vi "Min position limit.vi"(8 "error in (no error)":errorcluster, 9 "W/R":enum16{"Write", "Read"}(ring), 10 "Data":i32, 11 "Motor Base in":refnum<class "Motor Base.lvclass">) -> (0 "error out":errorcluster, 3 "Motor Base out":refnum<class "Motor Base.lvclass">)   [LabVIEW 2016, in "Motor Base.lvlib" / "Motor Base.lvclass"]
uses:
  Motor Base.lvclass
  Data Type.ctl
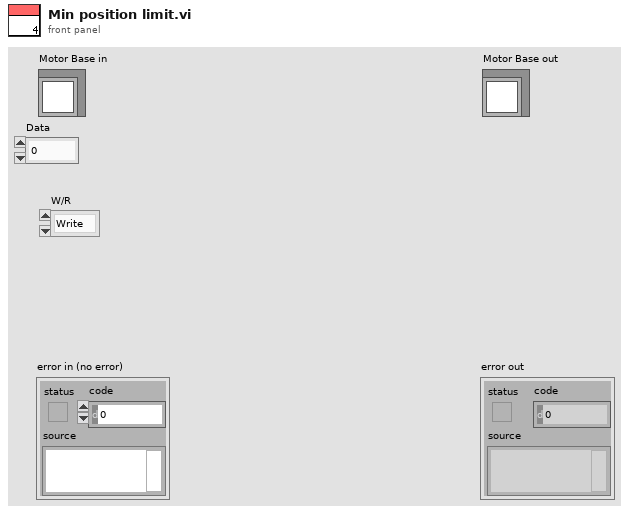
[diagram p1: front panel]
types:
  T1 = typedef "Motor Base.lvlib/Motor Base.lvclass/Data Type.ctl" = enum16{"BOOL", "I16", "I32", "I8", "OS", "U16", "U32", "U8", "VS"}
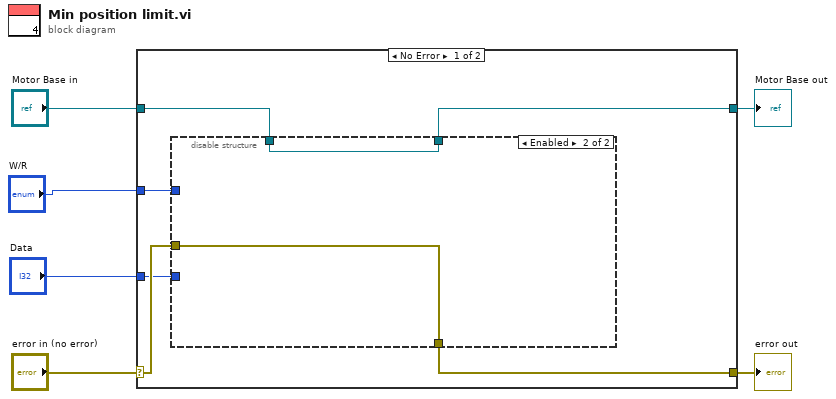
[diagram p0: block diagram]
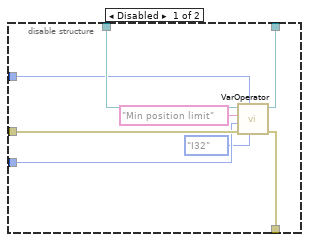
[diagram p2: hidden frame]
diagram:
  n1 = case shown="No Error" "error in (no error)" {
    selector: "error in (no error)" -> [w10 w24]
    tunnel: [w9 w24] -> w5
    tunnel: [w11 w23] -> w3
    tunnel: "Motor Base in" -> [w12 w23]
    tunnel: "Data" -> [w8 _]
    tunnel: "W/R" -> [w7 _]
    frame No Error {
      n2 = disable-structure shown="Enabled" {
        disable-tunnel: w12 -> [w20 w22]
        disable-tunnel: [w19 w22] -> w11
        disable-tunnel: w10 -> [w18 w21]
        disable-tunnel: [w17 w21] -> w9
        disable-tunnel: w8 -> [w15 _]
        disable-tunnel: w7 -> [w13 _]
        frame Disabled {
          n3 = call-dynamic "VarOperator.vi"("Data Type"=Data_Type."I32", "ro/w/r"=w13, "error in"=w18, "Data"=w15, "PDO Name"="Min position limit", "Motor Base in"=w20) -> ("error out"=w17:errorcluster, "Motor Base out"=w19:refnum<class "Motor Base.lvclass">)  [unwired: 1 in, 3 out]
        }
        frame Enabled {
        }
      }
    }
    frame Error {
    }
  }
  "error out" <- w5
  "Motor Base out" <- w3
